vi "Ctor.vi"(8 "error in (no error)":errorcluster, 11 "TCP Client in":refnum<class "TCP Client.lvclass">) -> (0 "error out":errorcluster, 3 "TCP Client out":refnum<class "TCP Client.lvclass">)   [LabVIEW 2020, in "Stream-TCP.lvlib" / "TCP Client.lvclass"]
uses:
  TCP Client.lvclass
  Client Command.ctl
  Ref Data.ctl
  TCP Stream/TCP Stream.lvclass
  Connection State.ctl
  TCP Mode.ctl
  TCP Client.lvclass/TCP Client.ctl
  lv-stream/stream/Connection/Connection.lvclass
  Stream-TCP.lvlib
  lv-trace/Trace/Trace.lvlib
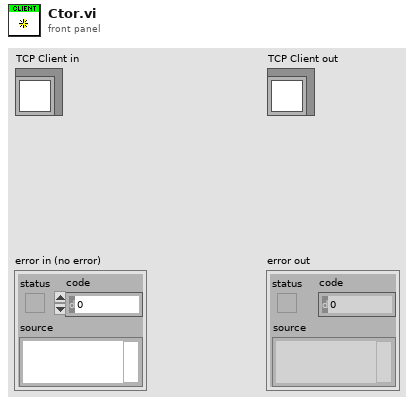
[diagram p1: front panel]
types:
  T1 = typedef "Stream-TCP.lvlib/TCP Mode.ctl" = enum16{"buffered", "raw"}
  T2 = typedef "Stream-TCP.lvlib/TCP Client.lvclass/Ref Data.ctl" = cluster{"TCP Connection":refnum<k5>, "TCP Stream":refnum<class "TCP Stream.lvclass">, "State":T3, "Connection Loop":refnum<vi>, "TCP Mode":T1, "Timeout ms":i32, "Server Connection":bool}
  T3 = typedef "Stream-TCP.lvlib/TCP Client.lvclass/Connection State.ctl" = enum16{"Closed", "Idle", "Connecting", "Connected", "Shutdown"}
  T4 = typedef "Stream-TCP.lvlib/Client Command.ctl" = enum16{"Connect", "Close", "Shutdown", "Reconnect"}
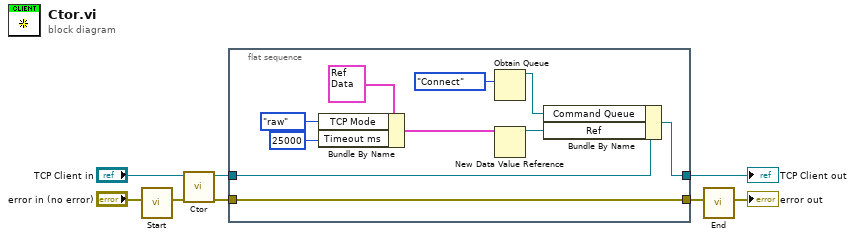
[diagram p0: block diagram]
diagram:
  n1 = call "Start.vi"("error in (no error)"="error in (no error)") -> ("error out"=w5:errorcluster)  [unwired: 10 in]
  n2 = call-parent "Ctor.vi"("error in (no error)"=w5, "Endpoint in"="TCP Client in") -> ("error out"=w2:errorcluster, "Endpoint out"=w3:refnum<class "TCP Client.lvclass">)  [unwired: 8 in]
  n3 = flat-sequence {
    tunnel: [w14] -> w8
    tunnel: w3 -> [w13]
    tunnel: w2 -> [w12]
    tunnel: [w12] -> w1
    frame #0 {
      n4 = Bundle By Name(cluster=T2 {"TCP Connection"=refnum, "TCP Stream"=refnum, "State"=enum."Closed", "Connection Loop"=refnum, "TCP Mode"=enum."buffered", "Timeout ms"=0, "Server Connection"=FALSE} ("Ref Data"), "TCP Mode"=TCP_Mode."raw", "Timeout ms"=25000) -> (w11:T2)
      n5 = Obtain Queue(element data type=Client_Command."Connect" ("Command")) -> (queue out=w15:refnum<queue>)  [unwired: 4 in, 2 out]
      n6 = New Data Value Reference(data value=w11) -> (data value reference=w17:refnum<data-value>)  [unwired: 1 in, 1 out]
      n7 = Bundle By Name(cluster=w13, "Command Queue"=w15, "Ref"=w17) -> (w14:refnum<class "TCP Client.lvclass">)
    }
  }
  n8 = call "End.vi"("error in (no error)"=w1) -> ("error out"=→"error out":errorcluster)  [unwired: 10 in]
  "TCP Client out" <- w8
